vi "Hall_custom functions.vi"(7 "Cluster":T3 caption="a1*FunctionA (a2*A)  (Operator)  b1*FunctionB (b2*B)", 10 "B":dbl[](array[numeric]), 11 "A":dbl[](array[numeric])) -> (0 "formula":string, 3 "result":dbl[](array[numeric]))   [LabVIEW 2025]
uses:
  controls/functions.ctl
  controls/operators.ctl
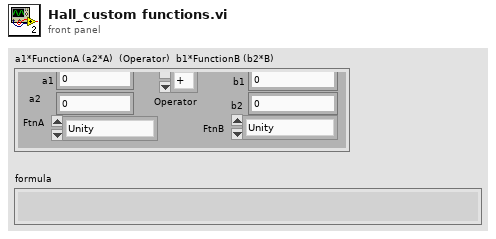
[diagram p1: front panel]
types:
  T1 = typedef "functions.ctl" = enum16{"Unity", "sin", "cos", "tan", "log10", "exp"}
  T2 = typedef "operators.ctl" = enum16{"+", "--", "*", "/"}
  T3 = cluster{"a1":dbl, "a2":dbl, "b1":dbl, "b2":dbl, "FtnA":T1, "Operator":T2, "FtnB":T1}
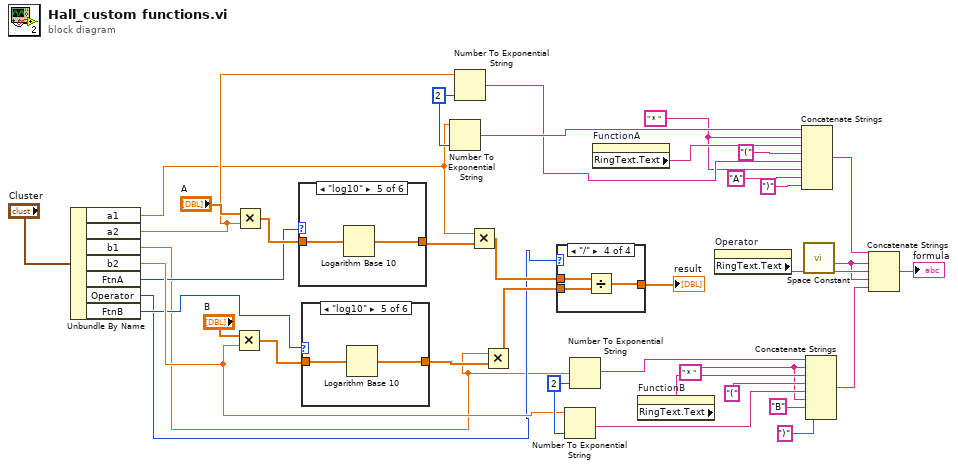
[diagram p0: block diagram]
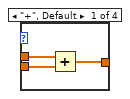
[diagram p2: hidden frame]
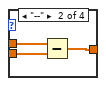
[diagram p3: hidden frame]
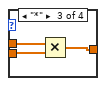
[diagram p4: hidden frame]
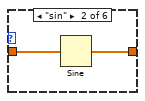
[diagram p6: hidden frame]
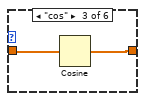
[diagram p7: hidden frame]
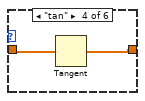
[diagram p8: hidden frame]
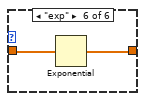
[diagram p9: hidden frame]
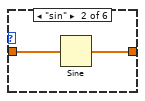
[diagram p11: hidden frame]
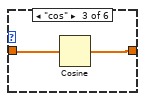
[diagram p12: hidden frame]
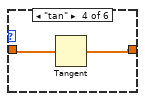
[diagram p13: hidden frame]
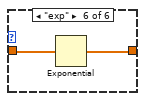
[diagram p14: hidden frame]
diagram:
  w9 = i16 2 ("precision (6)")
  w10 = i16 2 ("precision (6)")
  w18 = " * " ("string")
  w25 = " * " ("string")
  n1 = Unbundle By Name("Cluster") -> ("a1"=w2:dbl, "a2"=w7:dbl, "b1"=w1:dbl, "b2"=w6:dbl, "FtnA"=w5:T1, "Operator"=w3:T2, "FtnB"=w4:T1)
  n2 = Multiply(x="B", y=w6) -> (x*y=w35:dbl[])
  n3 = Multiply(x="A", y=w7) -> (x*y=w37:dbl[])
  n4 = case shown="\"log10\"" w5 {
    tunnel: w37 -> [w39 w41 w43 w45 w47 w49]
    tunnel: [w39 w40 w42 w44 w46 w48] -> w34
    frame "Unity", Default {
    }
    frame "sin" {
      n5 = Sine(x=w41) -> (sin(x)=w40:dbl[])
    }
    frame "cos" {
      n6 = Cosine(x=w43) -> (cos(x)=w42:dbl[])
    }
    frame "tan" {
      n7 = Tangent(1:w45) -> (0:w44:dbl[])
    }
    frame "log10" {
      n8 = Logarithm Base 10(1:w47) -> (0:w46:dbl[])
    }
    frame "exp" {
      n9 = Exponential(1:w49) -> (0:w48:dbl[])
    }
  }
  n10 = case shown="\"log10\"" w4 {
    tunnel: w35 -> [w50 w52 w54 w56 w58 w60]
    tunnel: [w50 w51 w53 w55 w57 w59] -> w33
    frame "Unity", Default {
    }
    frame "sin" {
      n11 = Sine(x=w52) -> (sin(x)=w51:dbl[])
    }
    frame "cos" {
      n12 = Cosine(x=w54) -> (cos(x)=w53:dbl[])
    }
    frame "tan" {
      n13 = Tangent(1:w56) -> (0:w55:dbl[])
    }
    frame "log10" {
      n14 = Logarithm Base 10(1:w58) -> (0:w57:dbl[])
    }
    frame "exp" {
      n15 = Exponential(1:w60) -> (0:w59:dbl[])
    }
  }
  n16 = Number To Exponential String(number=w2, precision (6)=w10) -> (E-format string=w29:string)  [unwired: 2 in]
  n17 = Number To Exponential String(number=w7, precision (6)=w10) -> (E-format string=w26:string)  [unwired: 2 in]
  n18 = Multiply(x=w2, y=w34) -> (x*y=w32:dbl[])
  n19 = Multiply(x=w1, y=w33) -> (x*y=w31:dbl[])
  n20 = case shown="\"/\"" w3 {
    tunnel: w32 -> [w63 w65 w69 w72]
    tunnel: w31 -> [w62 w66 w68 w71]
    tunnel: [w61 w64 w67 w70] -> w30
    frame "+", Default {
      n21 = Add(x=w63, y=w62) -> (x+y=w61:dbl[])
    }
    frame "--" {
      n22 = Subtract(x=w65, y=w66) -> (x-y=w64:dbl[])
    }
    frame "*" {
      n23 = Multiply(x=w69, y=w68) -> (x*y=w67:dbl[])
    }
    frame "/" {
      n24 = Divide(x=w72, y=w71) -> (x/y=w70:dbl[])
    }
  }
  "result" <- w30
  n25 = Number To Exponential String(number=w6, precision (6)=w9) -> (E-format string=w19:string)  [unwired: 2 in]
  n26 = Number To Exponential String(number=w1, precision (6)=w9) -> (E-format string=w22:string)  [unwired: 2 in]
  n27 = property on="FunctionA" class="Enum (strict)"() -> ("RingText.Text"=w28:string)  [unwired: 2 in, 2 out]
  n28 = property on="FunctionB" class="Enum (strict)"() -> ("RingText.Text"=w21:string)  [unwired: 2 in, 2 out]
  n29 = property on="Operator" class="Enum (strict)"() -> ("RingText.Text"=w14:string)  [unwired: 2 in, 2 out]
  n30 = Concatenate Strings(w29, w25, w28, "(" ("string"), w26, w25, "A" ("string"), ")" ("string")) -> (w15:string)
  n31 = call <vilib>:"Space Constant.vi"() -> ("String"=w13:string)
  n32 = Concatenate Strings(w22, w18, w21, "(" ("string"), w19, w18, "B" ("string"), ")" ("string")) -> (w12:string)
  n33 = Concatenate Strings(w15, w13, w14, w13, w12) -> (→"formula":string)
